vi "Voltage Diveder.vi"() -> (0 "VoltageOut":dbl)   [LabVIEW 2022 SP3]
panel:
  in  "R2":dbl
  in  "R1":dbl
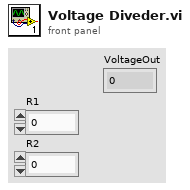
[diagram p1: front panel]
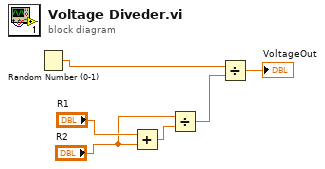
[diagram p0: block diagram]
diagram:
  n1 = Random Number (0-1)() -> (number: 0 to 1=w1:dbl)
  n2 = Add(x="R1", y="R2") -> (x+y=w4:dbl)
  n3 = Divide(x="R2", y=w4) -> (x/y=w3:dbl)
  n4 = Divide(x=w1, y=w3) -> (x/y=→"VoltageOut":dbl)
